vi "Test Humidity control.vi"() -> ()   [LabVIEW 2012]
uses:
  <vilib>/addons/control/pid/NI_PID_autopid.lvlib
  Reusable/General/Temperature/Temperature.lvlib
  Devices/Alicat/Data/MC/AlicatMCData.lvclass
  Reusable/General/Atmospheric/Atmospheric Library.lvlib
  Reusable/Data/Data.lvclass
panel:
  out "R":dbl=10000.000000163434 caption="R (Ohms)"
  in  "reinitialize? (F)":bool
  out "dt out (s)":dbl caption="Control\nLoop dt (s)" format="%.3f"
  in  "MFC SP":sgl[](array[numeric])=[0.16, 0.0, 0.0, 0.0, 3.0, 0.0, 0.0, 0.0, 0.0, 0.0]
  out "Array":T1(array[cluster])
  in  "Override":bool=TRUE
  in  "dt (s)":dbl=2.0 format="%.3f"
  in  "autotune? (F)":bool caption="Autotune"
  in  "PID gains init":T2={"proportional gain (Kc)"=0.1418303016781956, "integral time (Ti, min)"=4.732512769564583, "derivative time (Td, min)"=1.1831281923911459} caption="PID Parameters"
  out "timestamp":timestamp=timestamp(3396896939.1058674 s since 1904-01-01) format="%<%H:%M:%S%2u>T"
  in  "RHtarget":dbl=90.0 caption="RH (%)"
  in  "Vtec":dbl=1.6720317570902745 caption="TEC Voltage" min=0.0 max=6.0 step=0.01
  out "tecData":cluster{"Numeric":dbl, "Numeric":dbl}(graph)
  out "data":cluster{"[0]":dbl, "[1]":dbl, "[2]":dbl}(graph)
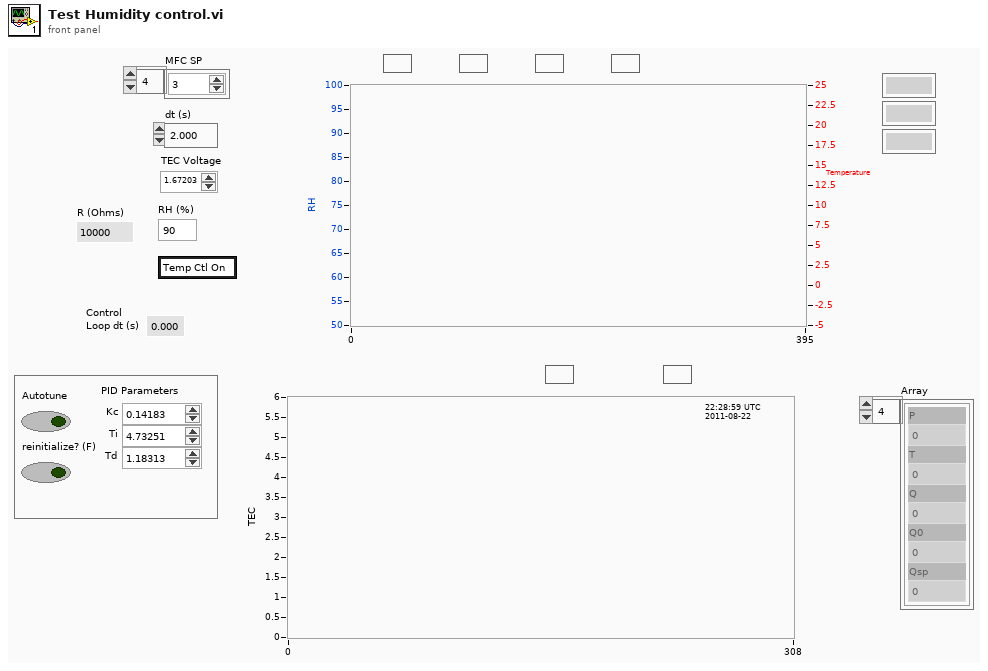
[diagram p1: front panel]
types:
  T1 = cluster{"P":sgl, "T":sgl, "Q":sgl, "Q0":sgl, "Qsp":sgl}[]
  T2 = cluster{"proportional gain (Kc)":dbl, "integral time (Ti, min)":dbl, "derivative time (Td, min)":dbl}
  T3 = cluster{"P":sgl, "T":sgl, "Q":sgl, "Q0":sgl, "Qsp":sgl}
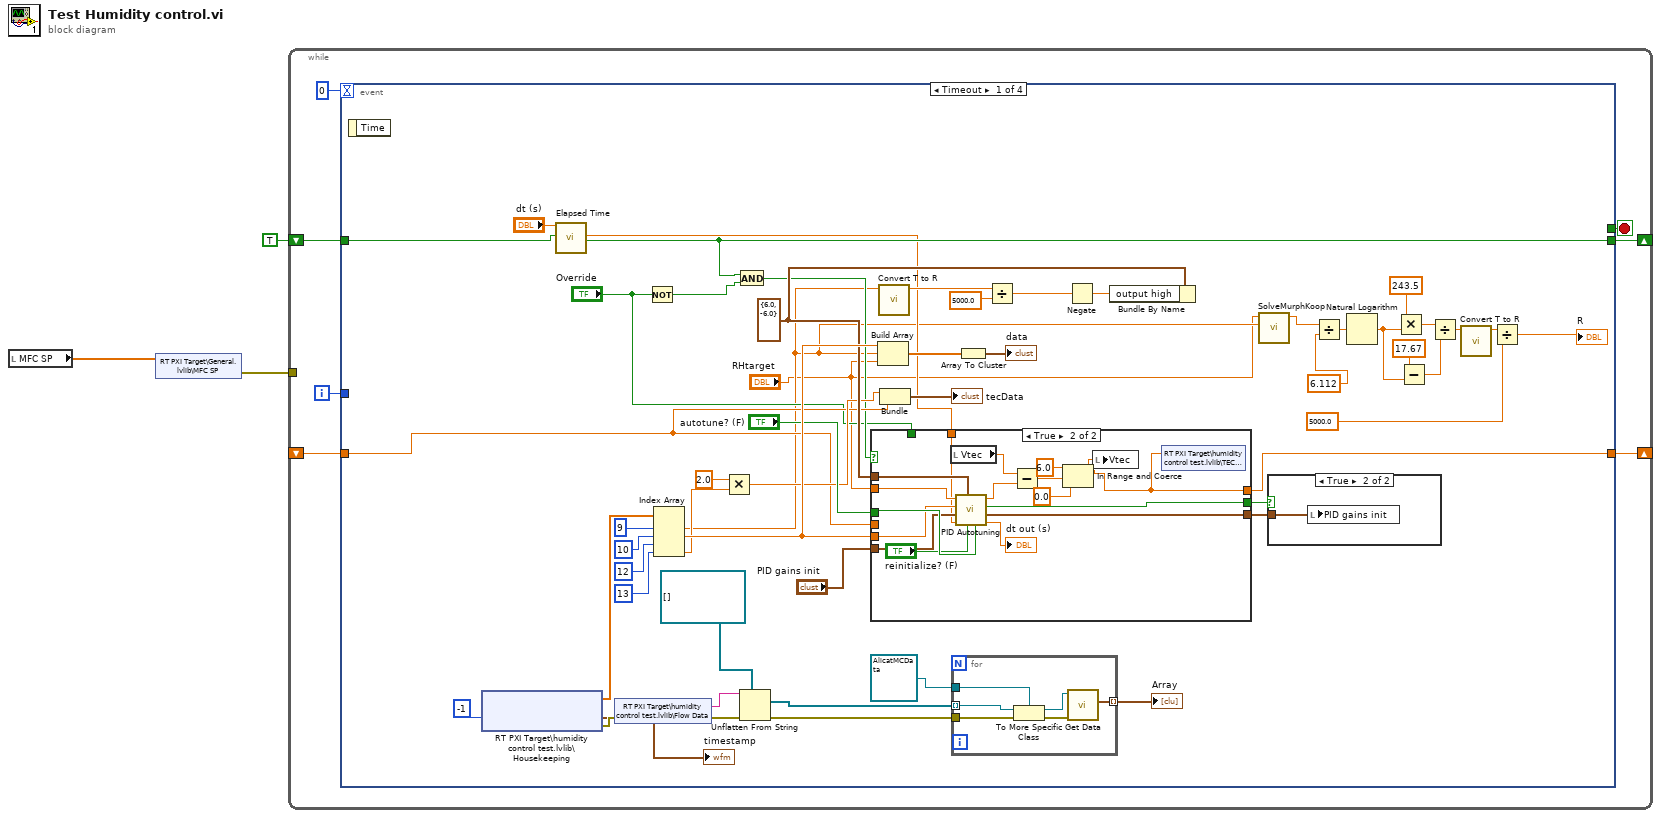
[diagram p0: block diagram]
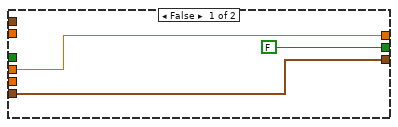
[diagram p2: hidden frame]
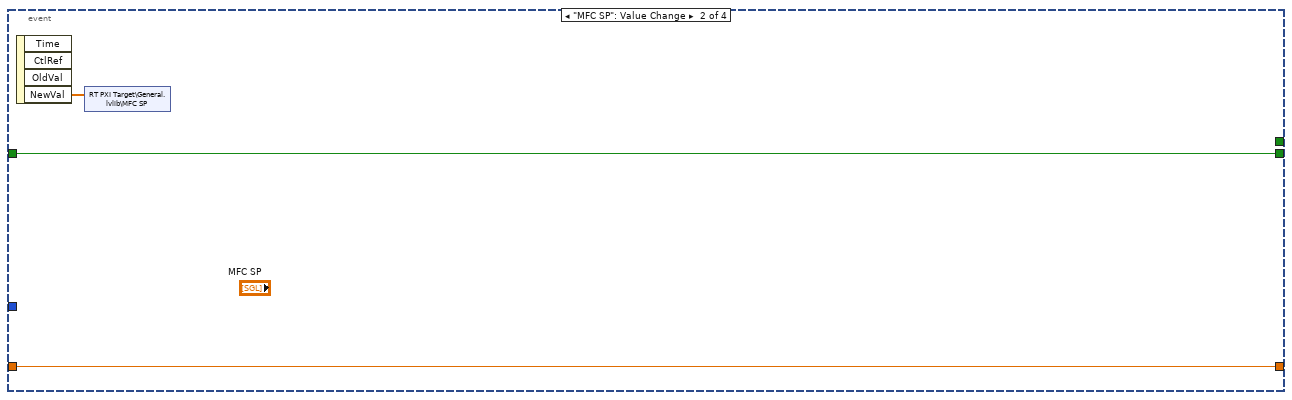
[diagram p4: hidden frame]
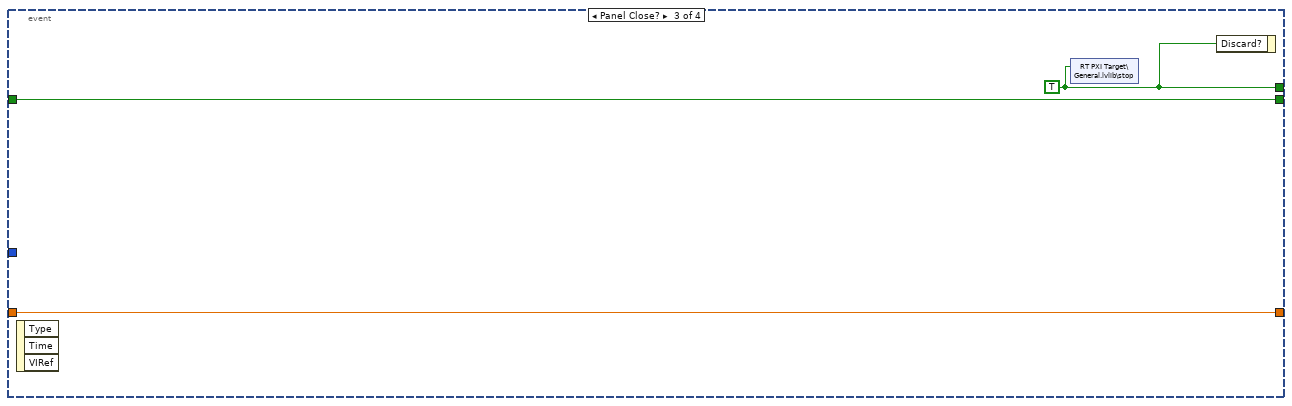
[diagram p5: hidden frame]
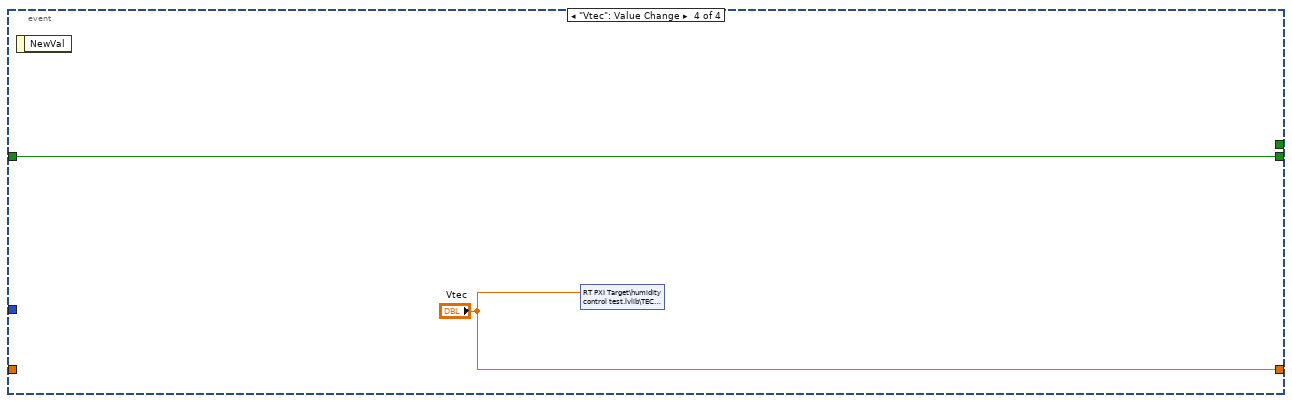
[diagram p6: hidden frame]
diagram:
  n1 = local read "MFC SP"() -> (w2:sgl[])
  n2 = shared-variable "RT PXI Target\\General.lvlib\\MFC SP"(w2) -> (error out=w1:errorcluster)  [unwired: 1 in]
  n3 = while {
    shift-right: [w7] -> _
    shift-left: TRUE ("Time has Elapsed") -> [w6]
    shift-right: [w5] -> _
    shift-left: _ -> [w4]
    tunnel: w1 -> [_]
    i -> [w8]
    stop <- w10 stop-if-true
    n4 = event shown="[0] Timeout" {
      selector: _ -> [_ _ _ _]
      dyn-events: _ -> [_ _ _ _]
      timeout: 0 -> [_ _ _ _]
      tunnel: [_ _ w96 _] -> w10
      tunnel: w8 -> [_ _ _ _]
      tunnel: [w32 w92 w94 w98] -> w7
      tunnel: w6 -> [w64 w92 w94 w98]
      tunnel: [w63 w93 w95 "Vtec"] -> w5
      tunnel: w4 -> [w27 w93 w95 _]
      event Timeout {
        w55 = cluster{"output high":dbl, "output low":dbl} {"output high"=6.0, "output low"=-6.0} ("output range")
        n5 = event-data() -> ()  [unwired: 1 in, 1 out]
        n6 = shared-variable "RT PXI Target\\humidity control test.lvlib\\Housekeeping"(-1 ("ms timeout (0)")) -> (w62:dbl[], error out=w51:errorcluster, →"timestamp":timestamp)  [unwired: 1 in, 1 out]
        n7 = call "Elapsed Time"("Time Target (s)"="dt (s)", "Reset"=w64) -> ("Elapsed Time (s)"=w31:dbl, "Time has Elapsed"=w32:bool)  [unwired: 10 in, 6 out]
        n8 = shared-variable "RT PXI Target\\humidity control test.lvlib\\Flow Data"(error in=w51) -> (w50:string, error out=w49:errorcluster)
        n9 = Not(x="Override") -> (.not. x?=w33:bool)
        n10 = Index Array(array=w62, index #1=9 ("index"), index #2=10 ("index"), index #3=12 ("index"), index #4=13 ("index")) -> (element #1=w24:dbl, element #2=w58:dbl, element #4=w30:dbl)  [unwired: 1 out]
        n11 = Multiply(x=2.0, y=w30) -> (x*y=w28:dbl)
        n12 = And(x=w32, y=w33) -> (x .and. y?=w26:bool)
        n13 = Unflatten From String(type=refnum<class "Data.lvclass">[] [], binary string=w50, error in (no error)=w49) -> (value=w47:refnum<class "Data.lvclass">[], error out=w46:errorcluster)  [unwired: 2 in, 1 out]
        n14 = case shown="True" w26 {
          tunnel: "autotune? (F)" -> [_ w83]
          tunnel: w55 -> [_ w82]
          tunnel: "RHtarget" -> [_ w81]
          tunnel: [w67 w68] -> w63
          tunnel: "PID gains init" -> [w65 w80]
          tunnel: [FALSE ("tuning completed?") w79] -> w41
          tunnel: [w65 w78] -> w40
          tunnel: w27 -> [w67 _]
          tunnel: w58 -> [_ w77]
          tunnel: w31 -> [_ w75]
          tunnel: "Override" -> [_ _]
          frame False {
          }
          frame True {
            n15 = local read "Vtec"() -> (w73:dbl)
            n16 = call <vilib>:"PID Autotuning.vi"("autotune? (F)"=w83, "reinitialize? (F)"="reinitialize? (F)", "output range"=w82, "dt (s)"=w75, "PID gains"=w80, "process variable"=w77, "setpoint"=w81) -> ("dt out (s)"=→"dt out (s)":dbl, "PID gains out"=w78:T2, "tuning completed?"=w79:bool, "output"=w72:dbl)  [unwired: 1 in]
            n17 = Subtract(x=w73, y=w72) -> (x-y=w71:dbl)
            n18 = In Range and Coerce(upper limit=6.0, x=w71, lower limit=0.0) -> (coerced(x)=w68:dbl)  [unwired: 1 out]
            n19 = local write "Vtec"(w68) -> ()
            n20 = shared-variable "RT PXI Target\\humidity control test.lvlib\\TEC_SP"(w68) -> ()  [unwired: 1 in, 1 out]
          }
        }
        n21 = Build Array(w58, w24, "RHtarget") -> (w57:dbl[])
        n22 = call "Convert T to R.vi"("T"=w24) -> ("R"=w39:dbl)  [unwired: 10 in]
        n23 = Bundle(w28, "Vtec"=w27) -> (→"tecData":cluster{dbl, "Vtec":dbl})  [unwired: 1 in]
        n24 = for {
          tunnel: w47 -> [w90] mode=indexing
          tunnel: w46 -> [w89]
          tunnel: refnum<class "AlicatMCData.lvclass"> refnum ("Alicat.lvlib:AlicatMCData.lvclass") -> [w88]
          tunnel: [w85] -> w44 mode=indexing
          n25 = To More Specific Class(target class=w88, reference=w90, error in=w89) -> (specific class reference=w87:refnum<class "AlicatMCData.lvclass">, error out=w86:errorcluster)
          n26 = call "Get Data.vi"("error in"=w86, "AlicatMData in"=w87) -> ("SystemData"=w85:T3)  [unwired: 7 in, 2 out]
        }
        "Array" <- w44
        n27 = Array To Cluster(array=w57) -> (cluster=→"data":cluster{"[0]":dbl, "[1]":dbl, "[2]":dbl})
        n28 = Divide(x=w39, y=5000.0) -> (x/y=w37:dbl)
        n29 = Negate(x=w37) -> (-x=w36:dbl)
        n30 = Bundle By Name(cluster=w55, "output high"=w36) -> ()  [unwired: 1 out]
        n31 = call "SolveMurphKoop.vi"("T"=w24, "RH"="RHtarget") -> ("e"=w12:dbl)  [unwired: 6 in, 3 out]
        n32 = case shown="True" w41 {
          tunnel: w40 -> [_ w84]
          frame False {
          }
          frame True {
            n33 = local write "PID gains init"(w84) -> ()
          }
        }
        n34 = Divide(x=w12, y=6.112) -> (x/y=w20:dbl)
        n35 = Natural Logarithm(1:w20) -> (0:w19:dbl)
        n36 = Multiply(x=243.5, y=w19) -> (x*y=w18:dbl)
        n37 = Subtract(x=17.67, y=w19) -> (x-y=w17:dbl)
        n38 = Divide(x=w18, y=w17) -> (x/y=w16:dbl)
        n39 = call "Convert T to R.vi"("T"=w16) -> ("R"=w15:dbl)  [unwired: 10 in]
        n40 = Divide(x=w15, y=5000.0) -> (x/y=→"R":dbl)
      }
      event "MFC SP": Value Change {
        n41 = event-data() -> ("NewVal"=w91:sgl[])  [unwired: 1 in, 3 out]
        n42 = shared-variable "RT PXI Target\\General.lvlib\\MFC SP"(w91) -> ()  [unwired: 1 in, 1 out]
      }
      event Panel Close? {
        w96 = TRUE ("Discard?")
        n43 = event-data() -> ()  [unwired: 1 in, 3 out]
        n44 = shared-variable "RT PXI Target\\General.lvlib\\stop"(w96) -> ()  [unwired: 1 in, 1 out]
        n45 = event-data("Discard?"=w96) -> ()  [unwired: 1 in, 1 out]
      }
      event "Vtec": Value Change {
        n46 = event-data() -> ()  [unwired: 1 in, 1 out]
        n47 = shared-variable "RT PXI Target\\humidity control test.lvlib\\TEC_SP"("Vtec") -> ()  [unwired: 1 in, 1 out]
      }
    }
  }
